vi "Set Fire Array.vi"(8 "error in (no error)":errorcluster, 9 "Duration (s)":dbl format="%#_13g", 10 "Fire (%)":dbl format="%#_13g", 11 "Cooker Actor in":refnum<class "Cooker Actor.lvclass">) -> (0 "error out":errorcluster, 3 "Cooker Actor out":refnum<class "Cooker Actor.lvclass">)   [LabVIEW 2024, in "Cooker Actor.lvlib" / "Cooker Actor.lvclass"]
uses:
  Cooker Actor.lvclass
  Cooker Actor.lvclass/Cooker Actor.ctl
  <vilib>/Analysis/NI_AALBase.lvlib
  <vilib>/Analysis/1siggen.llb/Ramp Pattern by Samples.vi
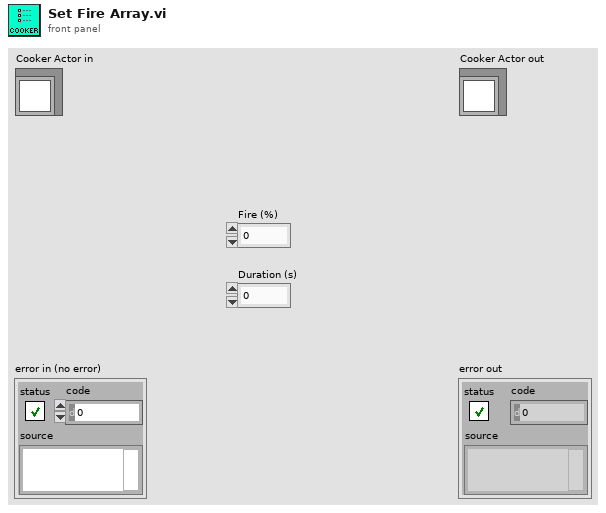
[diagram p1: front panel]
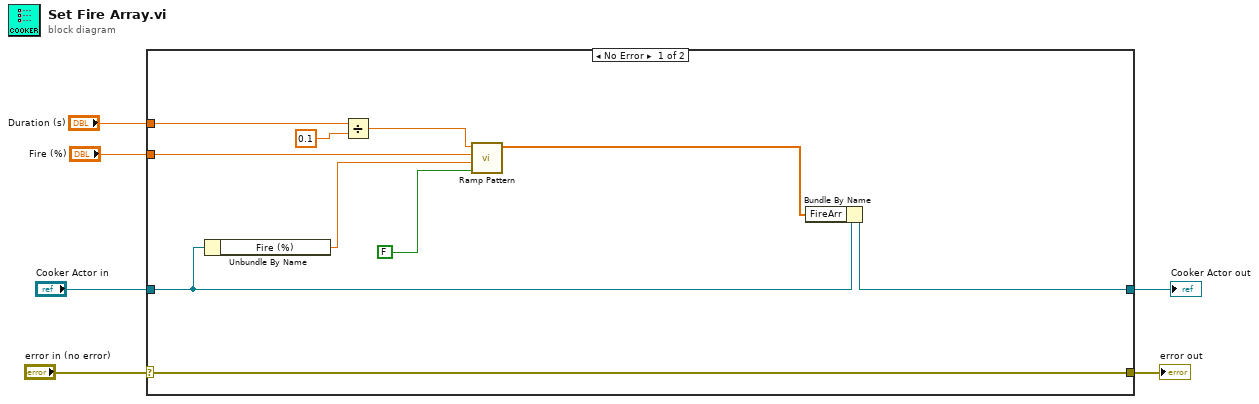
[diagram p0: block diagram]
diagram:
  n1 = case shown="No Error" "error in (no error)" {
    selector: "error in (no error)" -> [w16 w18]
    tunnel: [w16 w18] -> w5
    tunnel: [w8 w17] -> w3
    tunnel: "Cooker Actor in" -> [w15 w17]
    tunnel: "Fire (%)" -> [w14 _]
    tunnel: "Duration (s)" -> [w12 _]
    frame No Error {
      n2 = Unbundle By Name(w15) -> ("Fire (%)"=w10:dbl)
      n3 = Divide(x=w12, y=0.1) -> (x/y=w13:dbl)
      n4 = call-poly <vilib>:"Ramp Pattern.vi"("exclude end?"=FALSE, "start"=w10, "end"=w14, "samples"=w13) -> ("Ramp Pattern"=w7:dbl[])  [unwired: 6 in, 1 out]
      n5 = Bundle By Name(cluster=w15, "FireArr"=w7) -> (w8:refnum<class "Cooker Actor.lvclass">)
    }
    frame Error {
    }
  }
  "error out" <- w5
  "Cooker Actor out" <- w3
